vi "init.vi"(8 "error in (no error)":errorcluster, 9 "json of params":string, 10 "import":string, 11 "EnsembleBlender in":refnum<class "EnsembleBlender.lvclass">) -> (0 "error out":errorcluster, 3 "EnsembleBlender out":refnum<class "EnsembleBlender.lvclass">)   [LabVIEW 2020, in "EnsembleBlender.lvclass"]
uses:
  EnsembleBlender.lvclass
  C:/Users/cipop/TDF Dropbox/2_Technologies de France/1 - Services et Etudes/PLAIY/2 - DEV/PLAIYLAB/code/Python/Python.lvclass
  C:/Users/cipop/TDF Dropbox/2_Technologies de France/1 - Services et Etudes/PLAIY/2 - DEV/PLAIYLAB/code/Model/Model.lvclass
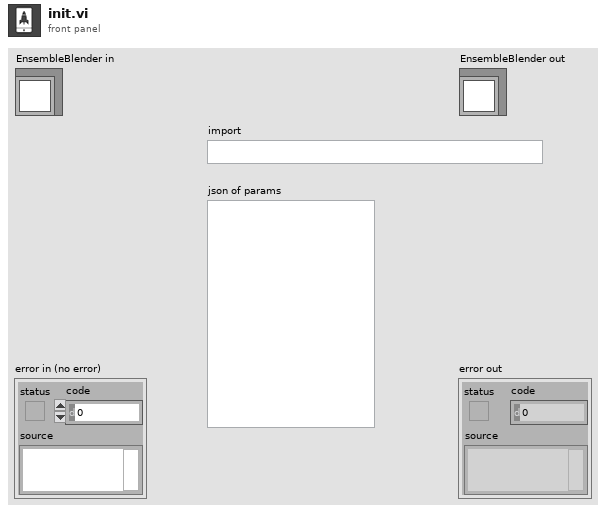
[diagram p1: front panel]
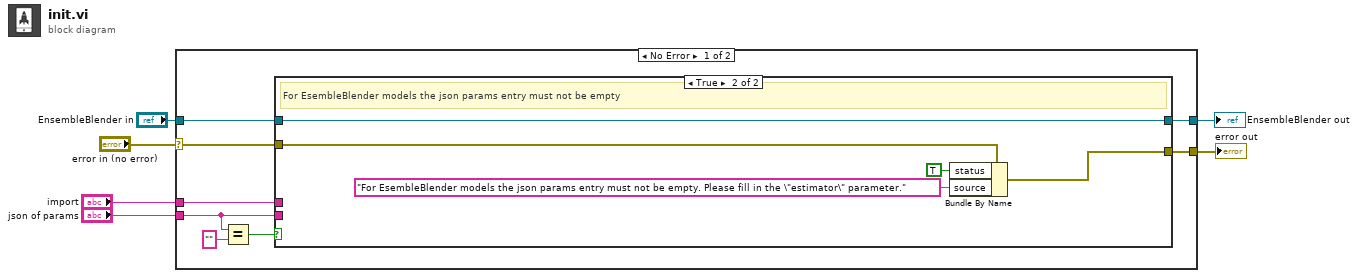
[diagram p0: block diagram]
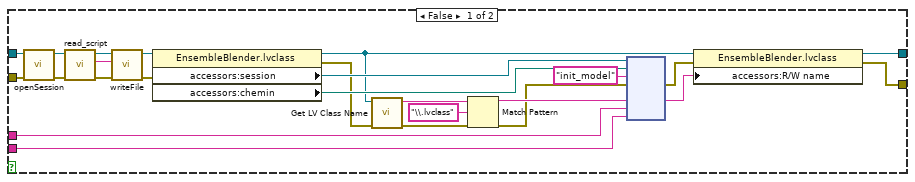
[diagram p2: hidden frame]
diagram:
  n1 = case shown="No Error" "error in (no error)" {
    selector: "error in (no error)" -> [w13 w45]
    tunnel: [w10 w45] -> w4
    tunnel: [w12 w44] -> w5
    tunnel: "EnsembleBlender in" -> [w14 w44]
    tunnel: "json of params" -> [w8 _]
    tunnel: "import" -> [w11 _]
    frame No Error {
      n2 = Equal?(x=w8, y="") -> (x = y?=w7:bool)
      n3 = case shown="True" w7 {
        tunnel: w14 -> [w38 w43]
        tunnel: w13 -> [w37 w39]
        tunnel: [w21 w43] -> w12
        tunnel: w11 -> [w18 _]
        tunnel: w8 -> [w17 _]
        tunnel: [w15 w42] -> w10
        frame False {
          n4 = call-dynamic "openSession.vi"("error in (no error)"=w37, "Python en entrée"=w38) -> ("error out"=w19:errorcluster, "Python en sortie"=w20:refnum<class "EnsembleBlender.lvclass">)  [unwired: 8 in]
          n5 = call-dynamic "read_script.vi"("error in (no error)"=w19, "Model en entrée"=w20) -> ("error out"=w34:errorcluster, "script"=w35:string, "Model en sortie"=w36:refnum<class "EnsembleBlender.lvclass">)  [unwired: 7 in]
          n6 = call-dynamic "writeFile.vi"("error in (no error)"=w34, "script"=w35, "Python en entrée"=w36) -> ("error out"=w31:errorcluster, "Python en sortie"=w32:refnum<class "EnsembleBlender.lvclass">)  [unwired: 7 in]
          n7 = property class="EnsembleBlender.lvclass"(reference=w32, error in=w31) -> (reference out=w23:refnum<class "EnsembleBlender.lvclass">, error out=w25:errorcluster, "accessors:session"=w30:refnum<k35>, "accessors:chemin"=w29:path)
          n8 = call <vilib>:"Get LV Class Name.vi"("error in (no error)"=w25, "object"=w23) -> ("error out"=w24:errorcluster, "class name"=w28:string)  [unwired: 8 in]
          n9 = Match Pattern(string=w28, regular expression="\\.lvclass") -> (before substring=w26:string)  [unwired: 1 in, 3 out]
          n10 = node(w30, w29, "init_model" ("nom de la fonction"), w24, w26, w18, w17) -> (w16:errorcluster, w22:string)  [unwired: 4 in, 3 out]
          n11 = property class="EnsembleBlender.lvclass"(reference=w23, error in=w16, "accessors:R/W name"=w22) -> (reference out=w21:refnum<class "EnsembleBlender.lvclass">, error out=w15:errorcluster)
        }
        frame True {
          # "For EsembleBlender models the json params entry must not be empty"
          n12 = Bundle By Name(cluster=w39, "status"=TRUE, "source"="For EsembleBlender models the json params entry must not be empty. Please fill in the \"estimator\" parameter.") -> (w42:errorcluster)
        }
      }
    }
    frame Error {
    }
  }
  "error out" <- w4
  "EnsembleBlender out" <- w5
